vi "Controle_leds_arrays.vi"() -> ()   [LabVIEW 2020]
panel:
  out "subarray":bool[](array[boolean])
  in  "Array":bool[][](array[boolean])
  in  "Comprimento de sequencia":i32
  out "LED 8":bool
  out "LED 7":bool
  out "LED 6":bool
  out "LED 5":bool
  out "LED 4":bool
  out "LED 3":bool
  out "LED 2":bool
  out "LED 1":bool
  in  "stop":bool
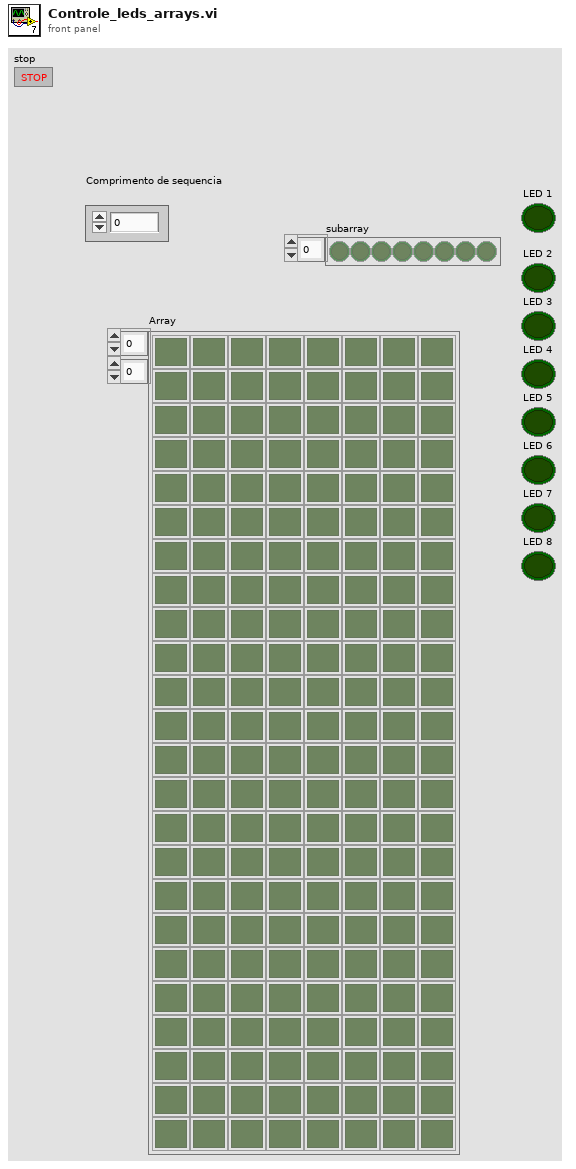
[diagram p1: front panel]
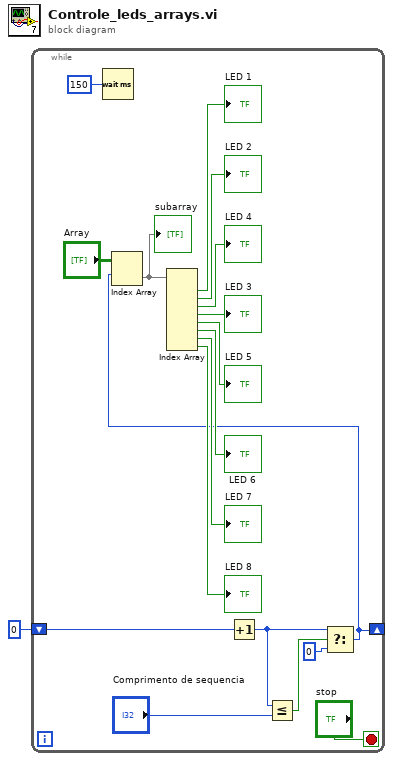
[diagram p0: block diagram]
diagram:
  n1 = while {
    shift-right: [w2] -> _
    shift-left: 0 -> [w6]
    stop <- "stop" stop-if-true
    n2 = Wait (ms)(milliseconds to wait=u32 150) -> ()  [unwired: 1 out]
    n3 = Increment(x=w6) -> (x+1=w5:i32)
    n4 = Less Or Equal?(x=w5, y="Comprimento de sequencia") -> (x <= y?=w4:bool)
    n5 = Select(t=w5, s=w4, f=0) -> (s? t:f=w2:i32)
    n6 = Index Array(array="Array", index (row)=w2) -> (element=w16:bool[])  [unwired: 1 in]
    "subarray" <- w16
    n7 = Index Array(array=w16) -> (element #1=→"LED 1":bool, element #2=→"LED 2":bool, element #3=→"LED 4":bool, element #4=→"LED 3":bool, element #5=→"LED 5":bool, element #6=→"LED 6":bool, element #7=→"LED 7":bool, element #8=→"LED 8":bool)  [unwired: 8 in]
  }
